vi "KPRO_2016_DPT.vi"() -> ()   [LabVIEW 2016]
uses:
  Kpro Globals.vi
  ad interface/Global_SIM_switch.vi
  <vilib>/Utility/file.llb/Write To Spreadsheet File (DBL).vi
panel:
  in  "Case Constant\n(See Context Help)":bool
  in  "Record DTW":bool
  out "Depth to Water":dbl=-30.877198474121087 format="%.2f"
  in  "In-Line Pressure Offset":dbl format="%.2f"
  in  "Zero In-Line Pressure\n(F = leave as is)":bool=TRUE
  in  "In-Line Pressure Slope":dbl=42.0 format="%.2f"
  out "In-Line Pressure":dbl=69.7228 format="%.2f"
  out "Drive Rate":dbl=16.666666666666664 format="%.2f"
  out "Real Time - Depth vs. Drive":cluster{dbl[], dbl[]}(graph)={[0.02036245163917736, 0.125, 0.16666666666666674, 0.16666666666666663, 0.16666666666666663, 0.16666666666666663], [-100.1, -100.2, -100.3, -100.4, -100.5, -100.6]}
  out "Current Depth (m)":sgl=-30.661383 format="%.2f"
  out "Zeroed \nPressure (m)":dbl=22.78027421497274 format="%.2f"
  out "Ik":dbl=0.003788962123473114 format="%.2f"
  in  "KPRO_test_report_header":string="Time(msecs)\tUncorrected_Depth\tCorrected_Depth\tDrive_Rate\tFlow\tFeet_of_Stainless\tPressure\tIK\tCorrected_Pressure\tAtm_Pressure\tDepth_to_water\tHeight_of_box\tRes_Pressure\tSecs_since_1_JAN_1904\tDepth_jumps_more_than_1_foot\r\n"
  in  "SLUG_test_report_header":string="Time(msecs)\tPressure\tFlow\n"
  in  "YSI_test_report_header":string="Depth\tPressure\tTemperature\tSpecific Conductivity\tDissolved O2\tPH\tOrp\tION\n"
  out "IK_for_GMS_report_header":string="Name\tHOLE_001\rXYZ\t20\t10\t30\rNumcols\t2\rNumrows\t1\rDepth\tIk\r"
  in  "Numrowswrite":string="1"
  in  "E":string="30"
  in  "Northing":string="10"
  in  "Easting":string="20"
  in  "Hole Id":string="HOLE_001"
  in  "Hole_name_file":path=path "C:/e"
  in  "Output File KPRO Test":path=path "C:/e_KPRO.txt"
  in  "Output File Slug Test":path=path "C:/e_SLUG.txt"
  in  "Output File YSI Test":path=path "C:/e_YSI.txt"
  in  "Output File IK for GMS":path=path "C:/e_IKMGS.txt"
  in  "enable_IKMGS_file":bool
  in  "enable_slug_file":bool
  in  "enable_kpro_file":bool=TRUE
  in  "enable_YSI_file":bool
  out "Ik":dbl=0.003788962123473114 format="%.2f"
  out "Zeroed Pressure":dbl=74.74207969932556 format="%.2f"
  out "Current Depth":sgl=-100.6 format="%.2f"
  out "Flow":dbl=0.21081600494384767 format="%.2f"
  out "Real Time - Depth vs. lk":cluster{dbl[], dbl[]}(graph)={[0.003788962123473114, 0.0037174584307500765, 0.0037174584307500765, 0.0037174584307500765, 0.0037174584307500765, 0.003788962123473114], [-100.1, -100.2, -100.3, -100.4, -100.5, -100.6]}
  out "Profile ID":string="WP-01"
  out "KPRO Box Number":dbl=800.0
  out "Last_String_Pot_Slope":dbl=1.6619999408721924 format="%.2f"
  out "Last_Flow_Slope":dbl=39.040000915527344 format="%.2f"
  out "Last_Pressure_Slope":dbl=48.27000045776367 format="%.2f"
  out "Height of Sample Box":dbl format="%.2f"
  out "Hole_Name_Path":path=path "C:/e"
  out "Cumulative_data_from_file":sgl[][](array[numeric]) format="%.2f"
  in  "data_directory":string="C:\\KPRO_DATA\\SITE_NAME\\"
  out "Cumulative_data_ready":bool
  out "Real Time - Depth vs. lk":cluster{dbl[], dbl[]}(graph)={[0.003788962123473114, 0.0037174584307500765, 0.0037174584307500765, 0.0037174584307500765, 0.0037174584307500765, 0.003788962123473114], [-100.1, -100.2, -100.3, -100.4, -100.5, -100.6]}
  in  "Reservoir Pressure":dbl=-0.004827000045779073 format="%.2f"
  in  "Simulate AD6B":bool
  in  "Atmospheric Pressure":dbl=32.22022530555725 format="%.2f"
  out "Depth to Water Table":dbl=-0.0 format="%.2f"
  in  "Ion Offset":dbl format="%.2f"
  in  "Ion Slope":dbl=44.04 format="%.2f"
  out "Pressure Slope":dbl=48.27000045776367 format="%.2f"
  out "Flow Slope":dbl=39.040000915527344 format="%.2f"
  out "String Pot Slope":dbl=1.6619999408721924 format="%.2f"
  in  "KPRO Com Port":i32=6
  in  "YSI Time Out (secs)":i32=5000
  in  "YSI Com Port":i32=7
  out "numrows":dbl format="%.2f"
  out "Slug Test\nIndicator copy":bool
  in  "ISE":bool=TRUE
  in  "Start\nYSI Capture":bool
  in  "Capture Head \nPressure":bool
  in  "Depth mode":bool caption="Use \nIncrement"
  out "Real Time - Depth vs. Drive":cluster{dbl[], dbl[]}(graph)={[0.02036245163917736, 0.125, 0.16666666666666674, 0.16666666666666663, 0.16666666666666663, 0.16666666666666663], [-100.1, -100.2, -100.3, -100.4, -100.5, -100.6]}
  out "Cumulative - Depth vs. Drive":cluster{dbl[], dbl[]}(graph)
  in  "Feet of Stainless":i32=40
  out "Zero Pressure\nIndicator":bool
  out "Slug Test\nIndicator":bool
  out "KPRO Test\nIndicator":bool
  in  "Increment\nButton":bool
  in  "Start\nST":bool
  in  "Zero\nPressure":bool
  out "Zeroed \nPressure":dbl=74.74207969932556 format="%.2f"
  in  "Finish Tests":bool
  out "Current Depth":sgl=-100.6 format="%.2f"
  in  "Start\nKPRO":bool
  out "Total Volume":dbl format="%.2f"
  in  "Clear \nTotal\nVolume":bool
  in  "Start Depth":sgl format="%.2f"
  in  "Client ID - Not Used":string
  out "Flow":dbl=0.21081600494384767 format="%.2f"
  out "Cumulative - Depth vs. Ik":cluster{dbl[], dbl[]}(graph)
  # "Use new slope/offset"
  # "KPRO  DATALOGGER"
  # "STONE  ENVIRONMENTAL  2010"
  # "ON"
  # "OFF"
  # "String Pot"
  # "Revision History\n\nAdded metric depth and pressure - VLD - 12-20-07\nAdded Static Ik button and drive rate- VLD 1-28-10"
  # "Use Incr"
  # "ON"
  # "OFF"
  # "ON"
  # "OFF"
  # "ON"
  # "OFF"
  # "ON"
  # "OFF"
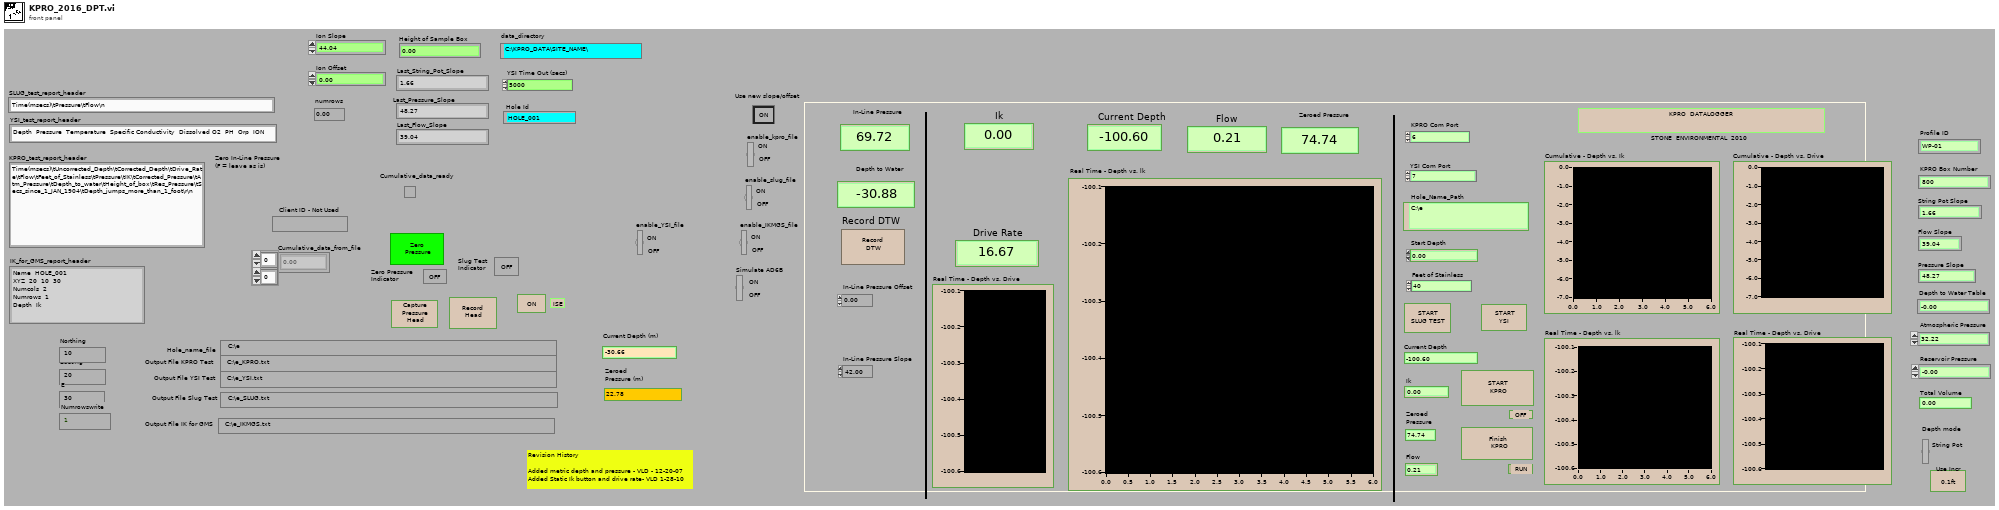
[diagram p1: front panel]
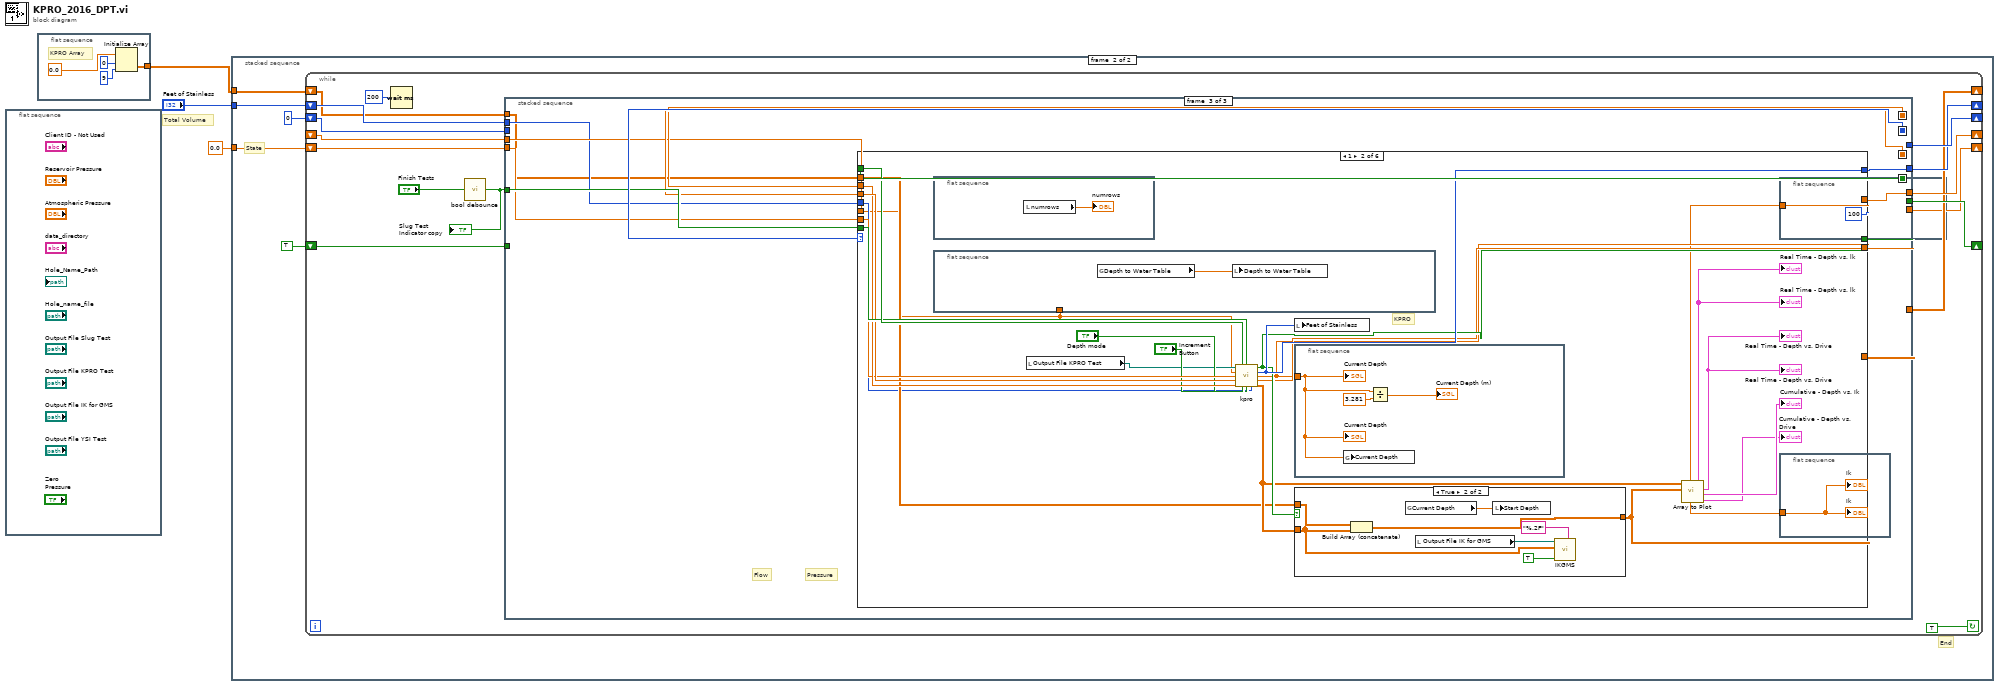
[diagram p0: block diagram]
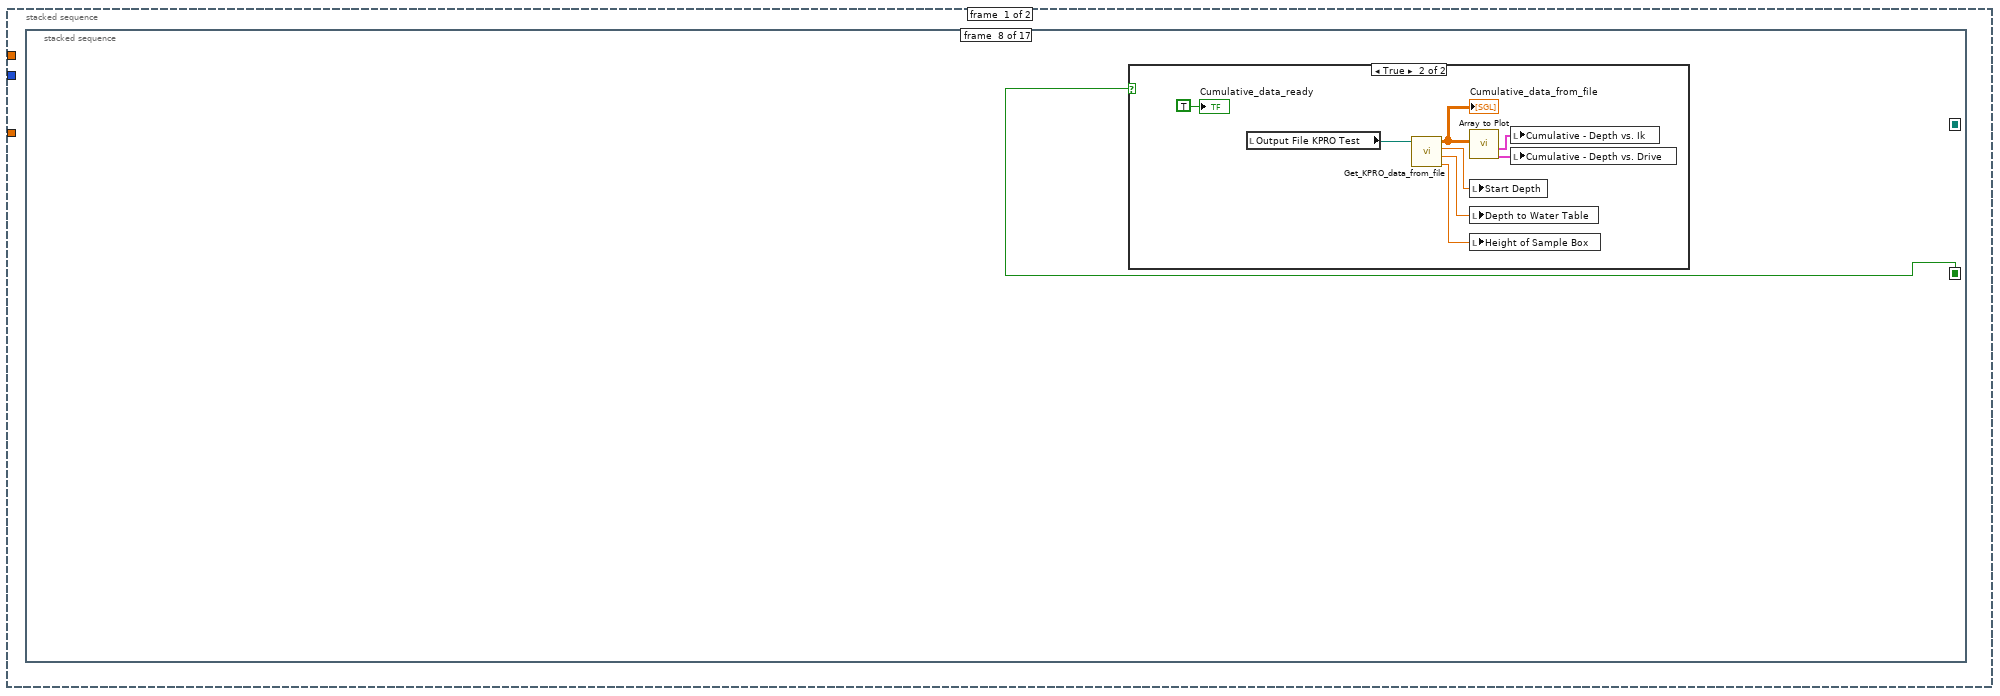
[diagram p2: hidden frame]
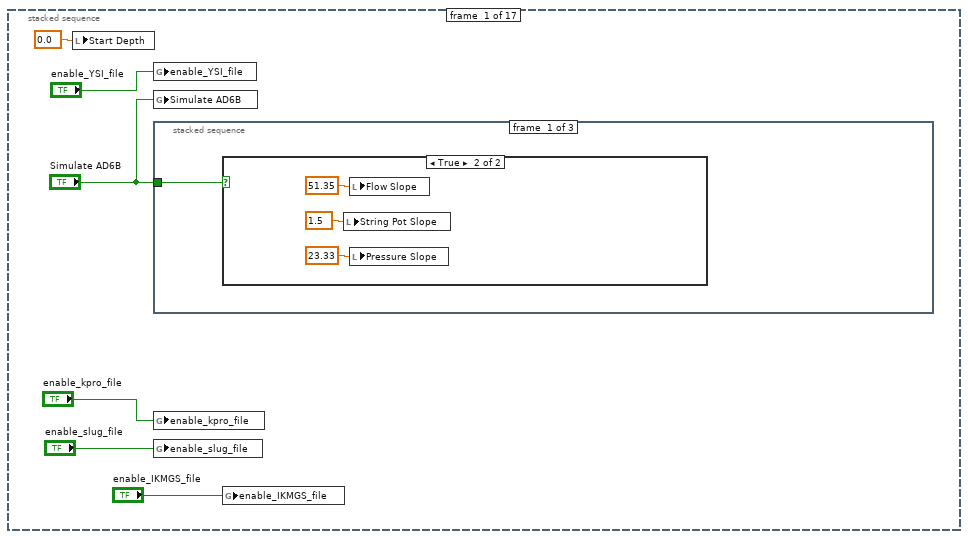
[diagram p3: hidden frame]
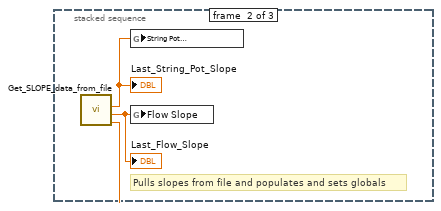
[diagram p5: hidden frame]
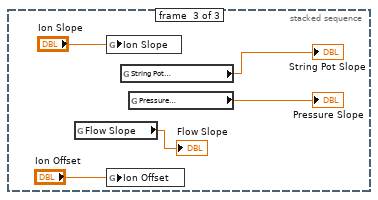
[diagram p6: hidden frame]
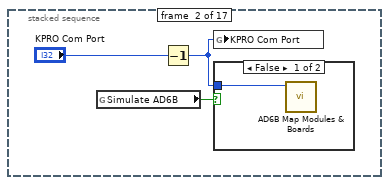
[diagram p7: hidden frame]
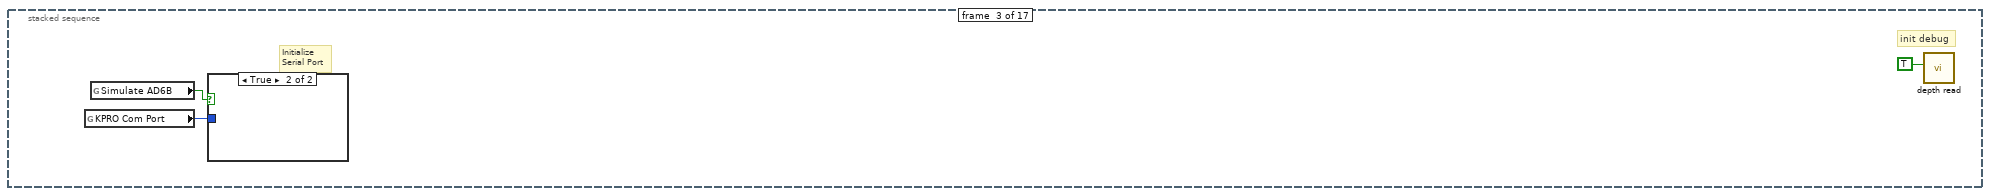
[diagram p9: hidden frame]
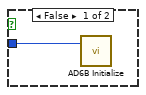
[diagram p10: hidden frame]
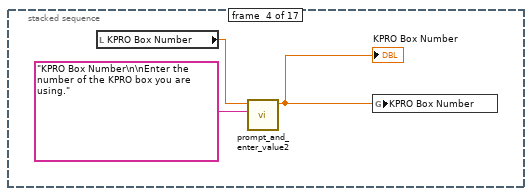
[diagram p11: hidden frame]
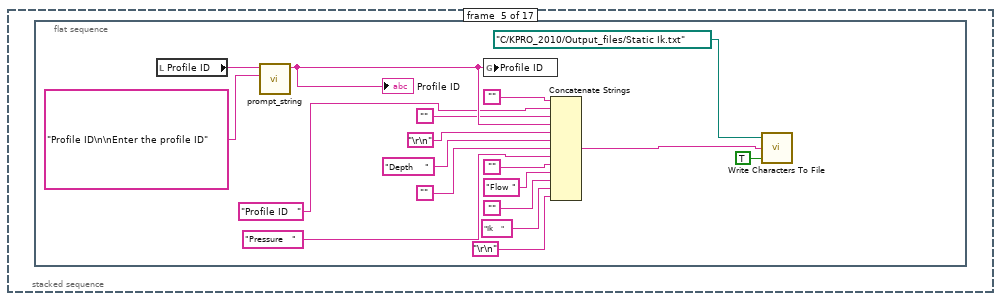
[diagram p12: hidden frame]
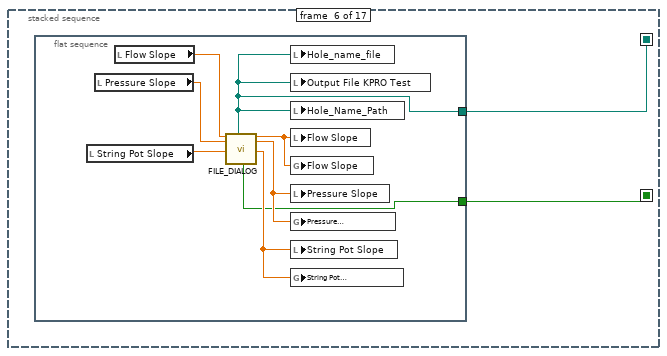
[diagram p13: hidden frame]
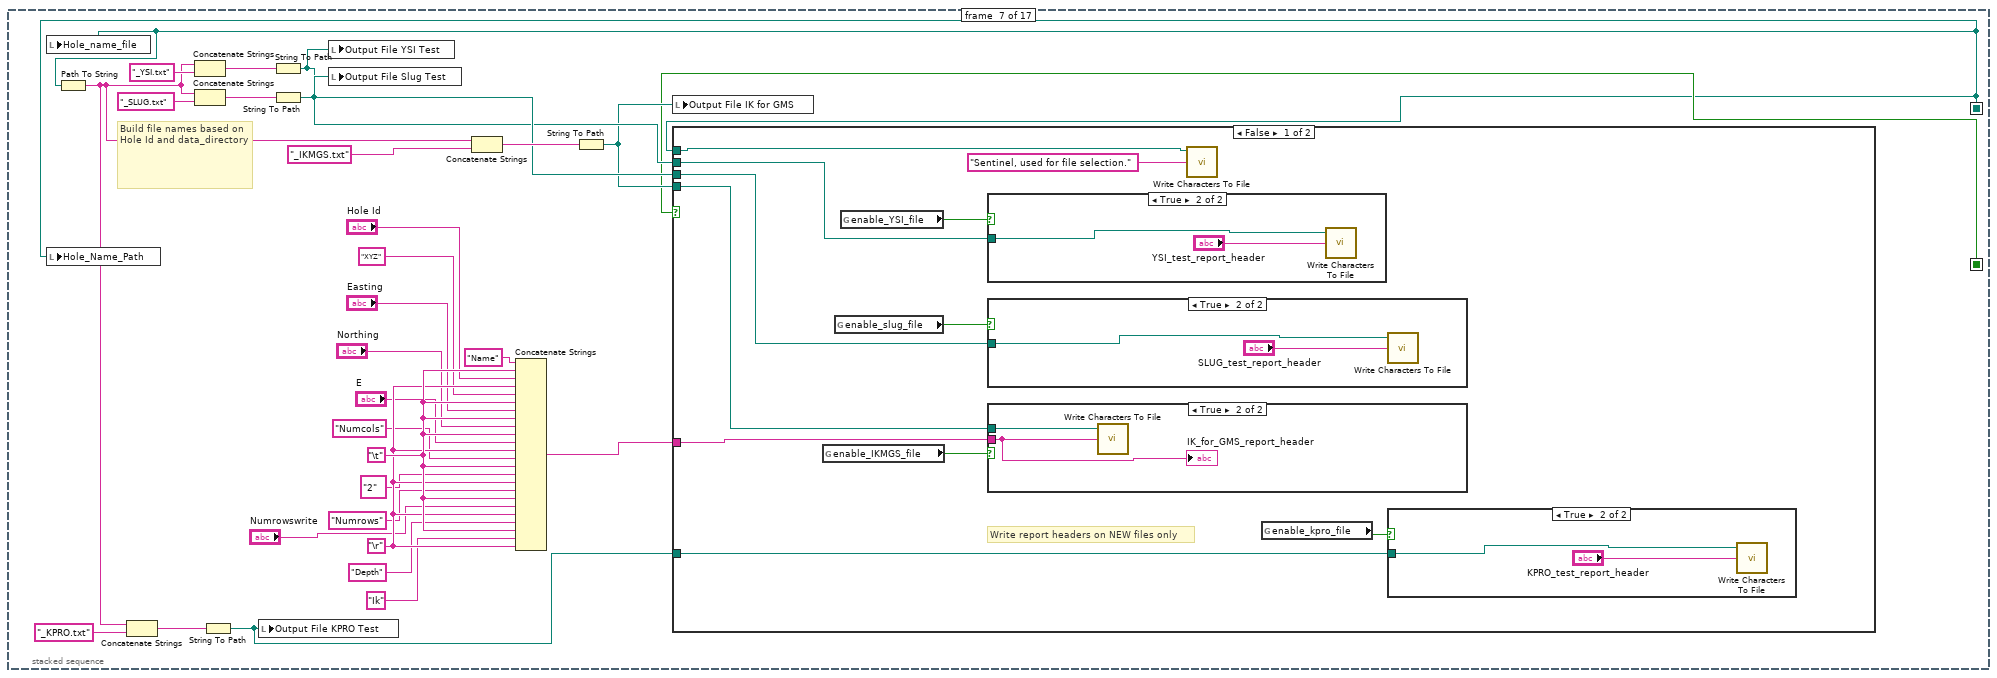
[diagram p14: hidden frame]
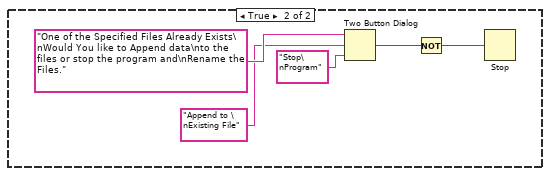
[diagram p19: hidden frame]
diagram:
  # "Total Volume"
  n1 = flat-sequence {
    frame #0 {
    }
  }
  n2 = flat-sequence {
    tunnel: [w4] -> w1
    frame #0 {
      # "KPRO Array"
      n3 = Initialize Array(0.0, 0, 9) -> (w4:dbl[][])
    }
  }
  n4 = stacked-sequence {
    tunnel: "Feet of Stainless" -> [_ w197]
    tunnel: 0.0 -> [_ w196]
    tunnel: w1 -> [_ w195]
    frame #0 {
      n5 = stacked-sequence {
        seq-local: [_ _ _ _ _ w55 _ _ _ _ _ _ _ _ _ _ _] -> [_ _ _ _ _ _ w66 w119 _ _ _ _ _ _ _ _ _]
        seq-local: [_ _ _ _ _ w56 _ _ _ _ _ _ _ _ _ _ _] -> [_ _ _ _ _ _ w65 _ _ _ _ _ _ _ _ _ _]
        frame #0 {
          n6 = local write "Start Depth"(sgl 0.0 ("Start Depth")) -> ()
          n7 = global write "Global_SIM_switch.vi" "enable_YSI_file"("enable_YSI_file") -> ()
          n8 = global write "Global_SIM_switch.vi" "Simulate AD6B"("Simulate AD6B") -> ()
          n9 = stacked-sequence {
            tunnel: "Simulate AD6B" -> [w14 _ _]
            frame #0 {
              n10 = case shown="True" w14 {
                frame False {
                }
                frame True {
                  n11 = local write "String Pot Slope"(1.5 ("String Pot Slope")) -> ()
                  n12 = local write "Flow Slope"(51.35 ("Flow Slope")) -> ()
                  n13 = local write "Pressure Slope"(23.33 ("Pressure Slope")) -> ()
                }
              }
            }
            frame #1 {
              # "Pulls slopes from file and populates and sets globals"
              n14 = call "Get_SLOPE_data_from_file.vi"() -> ("Last_Pressure_Slope"=w20:dbl, "Last_Flow_Slope"=w19:dbl, "Last_String_Pot_Slope"=w18:dbl)  [unwired: 8 in, 1 out]
              "Last_Pressure_Slope" <- w20
              "Last_Flow_Slope" <- w19
              "Last_String_Pot_Slope" <- w18
              n15 = global write "Kpro Globals.vi" "String Pot \nSlope"(w18) -> ()
              n16 = global write "Kpro Globals.vi" "Flow Slope"(w19) -> ()
              n17 = global write "Kpro Globals.vi" "Pressure \nSlope"(w20) -> ()
            }
            frame #2 {
              n18 = global read "Kpro Globals.vi" "Flow Slope"() -> (→"Flow Slope":dbl)
              n19 = global write "Kpro Globals.vi" "Ion Slope"("Ion Slope") -> ()
              n20 = global write "Kpro Globals.vi" "Ion Offset"("Ion Offset") -> ()
              n21 = global read "Kpro Globals.vi" "String Pot \nSlope"() -> (→"String Pot Slope":dbl)
              n22 = global read "Kpro Globals.vi" "Pressure \nSlope"() -> (→"Pressure Slope":dbl)
            }
          }
          n23 = global write "Global_SIM_switch.vi" "enable_kpro_file"("enable_kpro_file") -> ()
          n24 = global write "Global_SIM_switch.vi" "enable_slug_file"("enable_slug_file") -> ()
          n25 = global write "Global_SIM_switch.vi" "enable_IKMGS_file"("enable_IKMGS_file") -> ()
        }
        frame #1 {
          n26 = global read "Global_SIM_switch.vi" "Simulate AD6B"() -> (w26:bool)
          n27 = Decrement(x="KPRO Com Port") -> (x-1=w27:i32)
          n28 = global write "Kpro Globals.vi" "KPRO Com Port"(w27) -> ()
          n29 = case shown="False" w26 {
            tunnel: w27 -> [w29 _]
            frame False {
              n30 = call "AD6B Map Modules & Boards.VI"("port number (1:com2)"=w29) -> ()  [unwired: 3 in, 3 out]
            }
            frame True {
            }
          }
        }
        frame #2 {
          # "init debug"
          # "Initialize\nSerial Port"
          n31 = global read "Kpro Globals.vi" "KPRO Com Port"() -> (w30:i32)
          n32 = global read "Global_SIM_switch.vi" "Simulate AD6B"() -> (w31:bool)
          n33 = case shown="True" w31 {
            tunnel: w30 -> [w33 _]
            frame False {
              n34 = call "AD6B Initialize.VI"("port number (1:com2)"=w33) -> ()  [unwired: 2 in, 1 out]
            }
            frame True {
            }
          }
          n35 = call "depth read.vi"("Initialize Debug"=TRUE) -> ()  [unwired: 3 in, 1 out]
        }
        frame #3 {
          n36 = local read "KPRO Box Number"() -> (w34:dbl)
          n37 = call "prompt_and_enter_value2.vi"("prompt_IN"="KPRO Box Number\n\nEnter the number of the KPRO box you are using." ("prompt"), "Enter value"=w34) -> ("Numeric"=w35:dbl)  [unwired: 9 in]
          "KPRO Box Number" <- w35
          n38 = global write "Kpro Globals.vi" "KPRO Box Number"(w35) -> ()
        }
        frame #4 {
          n39 = flat-sequence {
            frame #0 {
              n40 = local read "Profile ID"() -> (w54:string)
              n41 = call "prompt_string.vi"("prompt_IN"="Profile ID\n\nEnter the profile ID" ("prompt"), "Enter value"=w54) -> ("String"=w50:string)  [unwired: 9 in]
              "Profile ID" <- w50
              n42 = global write "Kpro Globals.vi" "Profile ID"(w50) -> ()
              n43 = Concatenate Strings("" ("string"), "Profile ID   " ("string"), "" ("string"), w50, "\r\n", "Depth    " ("string"), "" ("string"), "Pressure   " ("string"), "" ("string"), "Flow " ("string"), "" ("string"), "Ik    " ("string"), "\r\n") -> (w49:string)
              n44 = call <vilib>:"Write Characters To File.vi"("append to file? (new file:F)"=TRUE, "character string"=w49, "file path (dialog if empty)"=path "C:/KPRO_2010/Output_files/Static Ik.txt") -> ()  [unwired: 2 in, 1 out]
            }
          }
        }
        frame #5 {
          n45 = flat-sequence {
            tunnel: [w58] -> w56
            tunnel: [w57] -> w55
            frame #0 {
              n46 = local read "String Pot Slope"() -> (w62:dbl)
              n47 = local read "Pressure Slope"() -> (w63:dbl)
              n48 = local read "Flow Slope"() -> (w64:dbl)
              n49 = call "FILE_DIALOG.vi"("flow_slope_IN"=w64, "pressure_slope_IN"=w63, "string_pot_slope_IN"=w62) -> ("path"=w58:path, "exists"=w57:bool, "flow_slope_OUT"=w61:dbl, "pressure_slope_OUT"=w60:dbl, "string_pot_slope_OUT"=w59:dbl)  [unwired: 9 in, 3 out]
              n50 = local write "Hole_name_file"(w58) -> ()
              n51 = local write "Output File KPRO Test"(w58) -> ()
              n52 = local write "Hole_Name_Path"(w58) -> ()
              n53 = local write "Flow Slope"(w61) -> ()
              n54 = global write "Kpro Globals.vi" "Flow Slope"(w61) -> ()
              n55 = local write "Pressure Slope"(w60) -> ()
              n56 = global write "Kpro Globals.vi" "Pressure \nSlope"(w60) -> ()
              n57 = local write "String Pot Slope"(w59) -> ()
              n58 = global write "Kpro Globals.vi" "String Pot \nSlope"(w59) -> ()
            }
          }
        }
        frame #6 {
          w94 = "\t"
          w93 = "\r" ("Carriage Return")
          # "Build file names based on Hole Id and data_directory"
          n59 = local write "Hole_name_file"(w65) -> ()
          n60 = local write "Hole_Name_Path"(w65) -> ()
          n61 = Path To String(path=w65) -> (string=w76:string)
          n62 = Concatenate Strings(w76, "_KPRO.txt") -> (w82:string)
          n63 = Concatenate Strings(w76, "_YSI.txt") -> (w80:string)
          n64 = Concatenate Strings(w76, "_SLUG.txt") -> (w81:string)
          n65 = String To Path(string=w82) -> (path=w75:path)
          n66 = local write "Output File KPRO Test"(w75) -> ()
          n67 = String To Path(string=w80) -> (path=w73:path)
          n68 = String To Path(string=w81) -> (path=w74:path)
          n69 = local write "Output File YSI Test"(w73) -> ()
          n70 = local write "Output File Slug Test"(w74) -> ()
          n71 = Concatenate Strings(w76, "_IKMGS.txt") -> (w79:string)
          n72 = Concatenate Strings("Name" ("Name"), w94, "Hole Id", w93, "XYZ" ("date string"), w94, "Easting", w94, "Northing", w94, "E", w93, "Numcols", w94, "2", w93, "Numrows", w94, "Numrowswrite", w93, "Depth", w94, "Ik", w93) -> (w85:string)
          n73 = String To Path(string=w79) -> (path=w72:path)
          n74 = local write "Output File IK for GMS"(w72) -> ()
          n75 = case shown="False" w66 {
            tunnel: w85 -> [w99 _]
            tunnel: w65 -> [w104 _]
            tunnel: w75 -> [w103 _]
            tunnel: w74 -> [w102 _]
            tunnel: w73 -> [w101 _]
            tunnel: w72 -> [w100 _]
            frame False {
              # "Write report headers on NEW files only"
              n76 = global read "Global_SIM_switch.vi" "enable_IKMGS_file"() -> (w95:bool)
              n77 = global read "Global_SIM_switch.vi" "enable_slug_file"() -> (w97:bool)
              n78 = global read "Global_SIM_switch.vi" "enable_YSI_file"() -> (w96:bool)
              n79 = case shown="True" w96 {
                tunnel: w101 -> [_ w109]
                frame False {
                }
                frame True {
                  n80 = call <vilib>:"Write Characters To File.vi"("character string"="YSI_test_report_header", "file path (dialog if empty)"=w109) -> ()  [unwired: 3 in, 1 out]
                }
              }
              n81 = case shown="True" w97 {
                tunnel: w102 -> [_ w111]
                frame False {
                }
                frame True {
                  n82 = call <vilib>:"Write Characters To File.vi"("character string"="SLUG_test_report_header", "file path (dialog if empty)"=w111) -> ()  [unwired: 3 in, 1 out]
                }
              }
              n83 = case shown="True" w95 {
                tunnel: w100 -> [_ w107]
                tunnel: w99 -> [_ w106]
                frame False {
                }
                frame True {
                  n84 = call <vilib>:"Write Characters To File.vi"("character string"=w106, "file path (dialog if empty)"=w107) -> ()  [unwired: 3 in, 1 out]
                  "IK_for_GMS_report_header" <- w106
                }
              }
              n85 = call <vilib>:"Write Characters To File.vi"("character string"="Sentinel, used for file selection.", "file path (dialog if empty)"=w104) -> ()  [unwired: 3 in, 1 out]
              n86 = global read "Global_SIM_switch.vi" "enable_kpro_file"() -> (w98:bool)
              n87 = case shown="True" w98 {
                tunnel: w103 -> [_ w113]
                frame False {
                }
                frame True {
                  n88 = call <vilib>:"Write Characters To File.vi"("character string"="KPRO_test_report_header", "file path (dialog if empty)"=w113) -> ()  [unwired: 3 in, 1 out]
                }
              }
            }
            frame True {
              n89 = Two Button Dialog(message="One of the Specified Files Already Exists\nWould You like to Append data\nto the files or stop the program and\nRename the Files.", 1:"Stop\nProgram", 2:"Append to \nExisting File") -> (T button?=w114:bool)
              n90 = Not(x=w114) -> (.not. x?=w115:bool)
              n91 = Stop(stop? (T)=w115) -> ()
            }
          }
        }
        frame #7 {
          n92 = case shown="True" w119 {
            frame False {
            }
            frame True {
              n93 = local read "Output File KPRO Test"() -> (w123:path)
              n94 = call "Get_KPRO_data_from_file.vi"("Output File KPRO Test"=w123) -> ("Last_height_of_box"=w120:dbl, "Last_depth_to_water"=w121:dbl, "Last_depth"=w127:dbl, "Output_array"=w124:sgl[][])  [unwired: 7 in]
              "Cumulative_data_from_file" <- w124
              n95 = call "Array to Plot.vi"("Input Cumulative Array"=w124) -> ("Cumulative - Depth vs.Drive Rate"=w125:cluster{dbl[], dbl[]}, "Cumulative - Depth vs. Ik"=w126:cluster{dbl[], dbl[]})  [unwired: 3 in, 4 out]
              n96 = local write "Start Depth"(w127) -> ()
              n97 = local write "Depth to Water Table"(w121) -> ()
              n98 = local write "Height of Sample Box"(w120) -> ()
              n99 = local write "Cumulative - Depth vs. Ik"(w126) -> ()
              n100 = local write "Cumulative - Depth vs. Drive"(w125) -> ()
              "Cumulative_data_ready" <- TRUE ("Cumulative_data_ready")
            }
          }
        }
        frame #8 {
          # "Start with Zero Offset for measurement of absolute pressure."
          n101 = global read "Global_SIM_switch.vi" "Simulate AD6B"() -> (w128:bool)
          n102 = case shown="False" w128 {
            tunnel: TRUE -> [w131 w133]
            tunnel: 0.0 -> [w132 w134]
            frame False {
              n103 = call "Pressure.vi"("Zero Pressure\n(F = leave as is)"=w131, "Pressure Offset"=w132) -> ()  [unwired: 1 in, 1 out]
            }
            frame True {
              n104 = call "SIM_Pressure.vi"("Zero Pressure\n(F = leave as is)"=w133, "Pressure Offset"=w134) -> ()  [unwired: 9 in, 1 out]
            }
          }
        }
        frame #9 {
          # "Take offset and put\n into Pressure VI."
          n105 = call "PRESSURE_CAL.vi"("sim_low"=29.9 ("sim_high"), "sim_high"=29.96, "Prompt_IN"="ATMOSPHERIC PRESSURE READING\n\nHold Kpro effluent facing up and level with the pressure transducer.\nTurn on Kpro water, turn off when water flows with no air bubbles.\n\nPress OK when the reading equilibrates." ("message")) -> ("PRESSURE\nFt of water"=w135:dbl)  [unwired: 8 in]
          n106 = global read "Global_SIM_switch.vi" "Simulate AD6B"() -> (w136:bool)
          n107 = global write "Kpro Globals.vi" "Atmospheric Pressure"(w135) -> ()
          n108 = local write "Atmospheric Pressure"(w135) -> ()
          n109 = case shown="False" w136 {
            tunnel: w135 -> [w142 w144]
            tunnel: TRUE -> [w141 w143]
            frame False {
              n110 = call "Pressure.vi"("Zero Pressure\n(F = leave as is)"=w141, "Pressure Offset"=w142) -> ()  [unwired: 1 in, 1 out]
            }
            frame True {
              n111 = call "SIM_Pressure.vi"("Zero Pressure\n(F = leave as is)"=w143, "Pressure Offset"=w144) -> ()  [unwired: 9 in, 1 out]
            }
          }
        }
        frame #10 {
          n112 = case shown="True" "Case Constant\n(See Context Help)" {
            frame False {
            }
            frame True {
              # "Take offset and put\n into Pressure VI."
              n113 = call "PRESSURE_CAL.vi"("sim_low"=30.9 ("sim_high"), "sim_high"=30.96, "Prompt_IN"="ZERO PRESSURE TRANSDUCER\n\nHold Kpro effluent in a grad cylinder with 800mL (1 ft) of water.\nHold grad cylinder with its bottom level with the pressure transducer.\n\nPress OK when the reading equilibrates. " ("message")) -> ("PRESSURE\nFt of water"=w146:dbl)  [unwired: 8 in]
              n114 = global read "Global_SIM_switch.vi" "Simulate AD6B"() -> (w148:bool)
              n115 = Subtract(x=w146, y=1.0) -> (x-y=w150:dbl)
              n116 = case shown="False" w148 {
                tunnel: [w155 w156] -> w149
                frame False {
                  n117 = call "Flow.vi"() -> ("Flow (ml/min)"=w155:dbl)  [unwired: 3 in]
                }
                frame True {
                  n118 = call "SIM_Flow.vi"() -> ("Flow (ml/min)"=w156:dbl)  [unwired: 3 in]
                }
              }
              n119 = case shown="False" w148 {
                tunnel: w150 -> [w158 w160]
                tunnel: TRUE -> [w157 w159]
                frame False {
                  n120 = call "Pressure.vi"("Zero Pressure\n(F = leave as is)"=w157, "Pressure Offset"=w158) -> ()  [unwired: 1 in, 1 out]
                }
                frame True {
                  n121 = call "SIM_Pressure.vi"("Zero Pressure\n(F = leave as is)"=w159, "Pressure Offset"=w160) -> ()  [unwired: 9 in, 1 out]
                }
              }
              n122 = local write "Flow"(w149) -> ()
            }
          }
        }
        frame #11 {
          n123 = call "PRESSURE_CAL.vi"("sim_low"=99.5 ("sim_high"), "sim_high"=100.5, "Prompt_IN"="CHECK RESERVOIR PRESSURE\n\nTurn on Kpro. Unplug Kpro Out quick connect from sample box.\nReservoir pressure should be 69.2 +/- 5%(65.7 - 72.7).\n\nPress OK when the reading equilibrates within range." ("message")) -> ("PRESSURE\nFt of water"=w163:dbl)  [unwired: 8 in]
          n124 = local write "Reservoir Pressure"(w163) -> ()
          n125 = global write "Kpro Globals.vi" "Reservoir Pressure"(w163) -> ()
        }
        frame #12 {
          n126 = local read "Start Depth"() -> (w169:sgl)
          n127 = call "prompt_and_enter_value 2016.vi"("prompt_IN"="ENTER START DEPTH", "Enter value"=w169) -> ("Numeric"=w167:dbl)  [unwired: 9 in]
          n128 = Absolute Value(x=w167) -> (abs(x)=w166:dbl)
          n129 = Negate(x=w166) -> (-x=w165:dbl)
          n130 = local write "Start Depth"(w165) -> ()
        }
        frame #13 {
          n131 = local read "Height of Sample Box"() -> (w171:dbl)
          n132 = call "prompt_and_enter_value 2016.vi"("prompt_IN"="HEIGHT FROM GROUND SURFACE TO SAMPLE BOX\n\nMeasure the vertical distance between the ground surface and the pressure transducer." ("prompt"), "Enter value"=w171) -> ("Numeric"=w170:dbl)  [unwired: 9 in]
          "Height of Sample Box" <- w170
          n133 = global write "Kpro Globals.vi" "height_of_box"(w170) -> ()
        }
        frame #14 {
          n134 = flat-sequence {
            frame #0 {
              n135 = local read "Depth to Water Table"() -> (w176:dbl)
              n136 = call "prompt_and_enter_value 2016.vi"("prompt_IN"="DEPTH TO WATER TABLE\n\nEnter the depth to the water table." ("prompt"), "Enter value"=w176) -> ("Numeric"=w175:dbl)  [unwired: 9 in]
              n137 = Absolute Value(x=w175) -> (abs(x)=w174:dbl)
              n138 = Negate(x=w174) -> (-x=w173:dbl)
              "Depth to Water Table" <- w173
              n139 = global write "Kpro Globals.vi" "Depth to Water Table"(w173) -> ()
            }
          }
        }
        frame #15 {
          n140 = stacked-sequence {
            frame #0 {
              # "Set to raw pressure mode"
              n141 = global read "Global_SIM_switch.vi" "Simulate AD6B"() -> (w179:bool)
              n142 = case shown="False" w179 {
                tunnel: TRUE -> [w180 w182]
                frame False {
                  n143 = call "Pressure.vi"("Zero Pressure\n(F = leave as is)"=w180, "Pressure Offset"=0.0) -> ()  [unwired: 1 in, 1 out]
                }
                frame True {
                  n144 = call "SIM_Pressure.vi"("Zero Pressure\n(F = leave as is)"=w182) -> ()  [unwired: 10 in, 1 out]
                }
              }
            }
            frame #1 {
              # "adjust for 1 foot head"
              # "Take offset and put\n into Pressure VI."
              n145 = global read "Global_SIM_switch.vi" "Simulate AD6B"() -> (w186:bool)
              n146 = call "PRESSURE_CAL.vi"("sim_low"=29.9 ("sim_high"), "sim_high"=29.96, "Prompt_IN"="ZERO TO GROUND SURFACE\n\nFill a grad cylinder to 750mL.\nPlace it on the ground at the profile location.\nImmerse the Kpro effluent and turn on Kpro flow.\nTurn off after water is flowing with no bubbles\nand the water has reached 800mL (1 foot).\n\nPress OK when the reading equilibrates." ("message")) -> ("PRESSURE\nFt of water"=w183:dbl)  [unwired: 8 in]
              n147 = Decrement(x=w183) -> (x-1=w184:dbl)
              n148 = case shown="False" w186 {
                tunnel: w184 -> [w191 w193]
                tunnel: TRUE -> [w190 w192]
                frame False {
                  n149 = call "Pressure.vi"("Zero Pressure\n(F = leave as is)"=w190, "Pressure Offset"=w191) -> ()  [unwired: 1 in, 1 out]
                }
                frame True {
                  n150 = call "SIM_Pressure.vi"("Zero Pressure\n(F = leave as is)"=w192, "Pressure Offset"=w193) -> ()  [unwired: 9 in, 1 out]
                }
              }
            }
          }
        }
        frame #16 {
          n151 = flat-sequence {
            frame #0 {
              w194 = FALSE
              n152 = local write "Slug Test\nIndicator"(w194) -> ()
              n153 = local write "KPRO Test\nIndicator"(w194) -> ()
              "Zero Pressure\nIndicator" <- w194
            }
          }
        }
      }
    }
    frame #1 {
      # "End"
      # "State"
      n154 = while {
        shift-left: w195 -> [w206]
        shift-right: [w205] -> _
        shift-left: w197 -> [w208]
        shift-right: [w207] -> _
        shift-left: _ -> [w211]
        shift-right: [w210] -> _
        shift-left: w196 -> [w209]
        shift-right: [w204] -> _
        shift-left: TRUE -> [w214]
        shift-right: [w213] -> _
        shift-left: 0 -> [w215]
        shift-right: [w212] -> _
        stop <- TRUE continue-if-true
        n155 = Wait (ms)(milliseconds to wait=u32 200) -> ()  [unwired: 1 out]
        n156 = call "bool debounce.vi"("Input Boolean"="Finish Tests") -> ("Output Boolean"=w202:bool)
        "Slug Test\nIndicator copy" <- w202
        n157 = stacked-sequence {
          seq-local: [_ w245 _] -> [_ _ w277]
          seq-local: [_ w256 _] -> [_ _ w276]
          seq-local: [w223 _ _] -> [_ _ w274]
          seq-local: [w224 _ _] -> [_ _ w273]
          tunnel: w215 -> [_ w258 _]
          tunnel: w214 -> [_ w257 _]
          tunnel: [_ _ w278] -> w213
          tunnel: [_ w245 _] -> w212
          tunnel: w202 -> [_ _ w275]
          tunnel: w211 -> [_ _ w272]
          tunnel: [_ _ w271] -> w210
          tunnel: w209 -> [_ _ w270]
          tunnel: [_ _ w269] -> w204
          tunnel: w208 -> [_ _ w268]
          tunnel: [_ _ w267] -> w207
          tunnel: w206 -> [_ _ w266]
          tunnel: [_ _ w265] -> w205
          frame #0 {
            n158 = global read "Kpro Globals.vi" "Current Depth"() -> (w219:sgl)
            n159 = call "In-Line-Pressure.vi"("Zero Pressure\n(F = leave as is)"="Zero In-Line Pressure\n(F = leave as is)", "In-Line Pressure Slope"="In-Line Pressure Slope", "In-Line Pressure Offset"="In-Line Pressure Offset") -> ("Pressure"=w220:dbl)  [unwired: 1 in]
            "In-Line Pressure" <- w220
            n160 = Add(x=w220, y=w219) -> (x+y=w216:dbl)
            "Depth to Water" <- w216
            n161 = case shown="True" "Record DTW" {
              selector: "Record DTW" -> [w230 _]
              tunnel: [w230 FALSE ("Boolean")] -> _
              tunnel: w216 -> [_ w234]
              tunnel: w219 -> [_ w235]
              tunnel: "In-Line Pressure Offset" -> [_ w232]
              tunnel: w220 -> [_ w233]
              tunnel: "In-Line Pressure Slope" -> [_ w231]
              frame False {
              }
              frame True {
                n162 = Build Array(w235, w234, w233, w232, w231) -> (w239:dbl[])
                n163 = call-poly <vilib>:"Write To Spreadsheet File.vi"("append to file? (new file:F)"=TRUE, "1D data"=w239, "file path (dialog if empty)"=path "C:/KPRO_2010/Output_files/DTW.txt") -> ()  [unwired: 5 in, 1 out]
              }
            }
            n164 = global read "Global_SIM_switch.vi" "Simulate AD6B"() -> (w225:bool)
            n165 = case shown="False" w225 {
              tunnel: [w242 w244] -> w224
              tunnel: [w241 w243] -> w223
              frame False {
                n166 = call "Flow.vi"() -> ("Flow (ml/min)"=w242:dbl)  [unwired: 3 in]
                n167 = call "Pressure.vi"("Zero Pressure\n(F = leave as is)"=FALSE ("Zero Pressure\n(F = leave as is)")) -> ("Pressure"=w241:dbl)  [unwired: 2 in]
              }
              frame True {
                n168 = call "SIM_Flow.vi"() -> ("Flow (ml/min)"=w244:dbl)  [unwired: 3 in]
                n169 = call "SIM_Pressure.vi"() -> ("Pressure"=w243:dbl)  [unwired: 11 in]
              }
            }
            n170 = flat-sequence {
              tunnel: w224 -> [w226]
              frame #0 {
                "Flow" <- w226
                "Flow" <- w226
              }
            }
            n171 = flat-sequence {
              tunnel: w223 -> [w229]
              frame #0 {
                n172 = Divide(x=w229, y=3.281) -> (x/y=→"Zeroed \nPressure (m)":dbl)
                "Zeroed \nPressure" <- w229
                "Zeroed Pressure" <- w229
              }
            }
          }
          frame #1 {
            n173 = call "State Controller.vi"("Start KPRO"="Start\nKPRO", "Start Slug Test"="Start\nST", "Start YSI Capture"="Start\nYSI Capture", "Clear Volume"="Clear \nTotal\nVolume", "Capture Head Pressure"="Capture Head \nPressure", "Done"=w257, "Previous \nState"=w258) -> ("Next State"=w245:i32, "State Changed"=w256:bool, "Start KPRO Enabler"=w250:u8, "Start Slug Test Enabler"=w249:u8, "Start YSI Capture Enabler"=w248:u8, "Clear Volume Enabler"=w247:u8, "Capture Head Pressure Enabler"=w246:u8)  [unwired: 4 in, 2 out]
            n174 = property on="Start\nKPRO" class="Bool"("Disabled"=w250) -> ()  [unwired: 2 in, 2 out]
            n175 = property on="Start\nST" class="Bool"("Disabled"=w249) -> ()  [unwired: 2 in, 2 out]
            n176 = property on="Clear \nTotal\nVolume" class="Bool"("Disabled"=w247) -> ()  [unwired: 2 in, 2 out]
            n177 = flat-sequence {
              tunnel: w245 -> [w259]
              frame #0 {
                n178 = Equal?(x=w259, y=2) -> (x = y?=→"Slug Test\nIndicator":bool)
              }
            }
            n179 = flat-sequence {
              tunnel: w245 -> [w262]
              frame #0 {
                n180 = Equal?(x=w262, y=1) -> (x = y?=→"KPRO Test\nIndicator":bool)
              }
            }
            n181 = property on="Start\nYSI Capture" class="Bool"("Disabled"=w248) -> ()  [unwired: 2 in, 2 out]
            n182 = property on="Capture Head \nPressure" class="Bool"("Disabled"=w246) -> ()  [unwired: 2 in, 2 out]
          }
          frame #2 {
            # "Flow"
            # "Pressure"
            n183 = case shown="1" w277 {
              tunnel: [FALSE w307 w333 w340 TRUE TRUE] -> w278
              tunnel: w276 -> [_ w315 w333 w342 _ _]
              tunnel: w275 -> [_ w314 _ w341 _ _]
              tunnel: w274 -> [_ w313 _ _ _ w361]
              tunnel: w273 -> [_ w312 _ _ _ _]
              tunnel: w272 -> [_ w293 w334 w343 w358 w360]
              tunnel: [w279 w297 w334 w343 w358 w360] -> w271
              tunnel: w270 -> [w284 w311 w337 w346 _ w365]
              tunnel: [w284 w302 w337 w346 0.0 w365] -> w269
              tunnel: w268 -> [w283 w294 w335 w345 w356 w364]
              tunnel: [w283 w308 w335 w345 w356 w364] -> w267
              tunnel: w266 -> [w282 w301 w336 w344 w355 w363]
              tunnel: [w281 w305 w336 w344 w355 w363] -> w265
              frame 0, Default {
                # "Idle State"
                n184 = local read "Cumulative_data_ready"() -> (w280:bool)
                n185 = case shown="True" w280 {
                  tunnel: w282 -> [w290 _]
                  tunnel: [w290 w291] -> w281
                  frame False {
                  }
                  frame True {
                    n186 = local read "Cumulative_data_from_file"() -> (w291:sgl[][])
                    n187 = local write "Cumulative_data_ready"(FALSE ("Get_KPRO_data")) -> ()
                  }
                }
                n188 = flat-sequence {
                  tunnel: [w286] -> w279
                  frame #0 {
                    n189 = Less Or Equal To 0?(x="Start Depth") -> (x <= 0?=w289:bool)
                    n190 = Negate(x="Start Depth") -> (-x=w287:sgl)
                    n191 = Select(t="Start Depth", s=w289, f=w287) -> (s? t:f=w286:sgl)
                  }
                }
              }
              frame 1 {
                # "KPRO"
                n192 = flat-sequence {
                  frame #0 {
                    n193 = local read "numrows"() -> (→"numrows":dbl)
                  }
                }
                n194 = flat-sequence {
                  tunnel: w293 -> [_]
                  frame #0 {
                    n195 = global read "Kpro Globals.vi" "Depth to Water Table"() -> (w317:dbl)
                    n196 = local write "Depth to Water Table"(w317) -> ()
                  }
                }
                n197 = local read "Output File KPRO Test"() -> (w300:path)
                n198 = call "kpro.vi"("Output KPRO"=w300, "Initialize"=w315, "Finished In"=w314, "Absolute Depth In"=w293, "Total Volume in"=w311, "Zeroed Pressure"=w313, "Flow"=w312, "Read String Pot"="Depth mode", "Increment"="Increment\nButton", "SS In"=w294) -> ("Finished Out"=w307:bool, "SS Out"=w308:i32, "Current Depth Out"=w297:sgl, "Total Volume Out"=w302:dbl, "Output Array"=w306:dbl[][])  [unwired: 1 in]
                n199 = local write "Feet of Stainless"(w308) -> ()
                n200 = flat-sequence {
                  tunnel: w297 -> [w320]
                  frame #0 {
                    n201 = global write "Kpro Globals.vi" "Current Depth"(w320) -> ()
                    n202 = Divide(x=w320, y=3.281) -> (x/y=→"Current Depth (m)":dbl)
                    "Current Depth" <- w320
                    "Current Depth" <- w320
                  }
                }
                n203 = case shown="True" w307 {
                  tunnel: [w325 w332] -> w305
                  tunnel: w306 -> [_ w331]
                  tunnel: w301 -> [w325 w327]
                  frame False {
                  }
                  frame True {
                    n204 = Build Array (concatenate)(w327, w331) -> (w332:dbl[][])
                    n205 = global read "Kpro Globals.vi" "Current Depth"() -> (w326:sgl)
                    n206 = local read "Output File IK for GMS"() -> (w329:path)
                    n207 = local write "Start Depth"(w326) -> ()
                    n208 = call "IKGMS.vi"("format (%.3f)"="%.2F", "append to file? (new file:F)"=TRUE, "2D data"=w331, "file path (dialog if empty)"=w329) -> ()  [unwired: 4 in, 1 out]
                  }
                }
                n209 = call "Array to Plot.vi"("Input Cumulative Array"=w305, "Input Real Time Array"=w306) -> ("Cumulative - Depth vs.Drive Rate"=→"Cumulative - Depth vs. Drive":cluster{dbl[], dbl[]}, "Cumulative - Depth vs. Ik"=→"Cumulative - Depth vs. Ik":cluster{dbl[], dbl[]}, "Real Time - Depth vs. Drive Rate"=→"Real Time - Depth vs. Drive" →"Real Time - Depth vs. Drive":cluster{dbl[], dbl[]}, "Real Time - Depth vs. Ik"=→"Real Time - Depth vs. lk" →"Real Time - Depth vs. lk":cluster{dbl[], dbl[]}, "Current Ik"=w296:dbl, "Depth Rate"=w295:dbl)  [unwired: 2 in]
                n210 = flat-sequence {
                  tunnel: w295 -> [w323]
                  frame #0 {
                    n211 = Multiply(x=w323, y=100) -> (x*y=→"Drive Rate":dbl)
                  }
                }
                n212 = flat-sequence {
                  tunnel: w296 -> [w316]
                  frame #0 {
                    "Ik" <- w316
                    "Ik" <- w316
                  }
                }
              }
              frame 2 {
                n213 = flat-sequence {
                  tunnel: w335 -> [w339]
                  frame #0 {
                    n214 = local read "Output File Slug Test"() -> (w338:path)
                    n215 = call "Slug Test.vi"("# SS"=w339, "Output File"=w338) -> ()  [unwired: 10 in]
                  }
                }
              }
              frame 3 {
                n216 = flat-sequence {
                  tunnel: w343 -> [w353]
                  tunnel: w342 -> [w352]
                  tunnel: w341 -> [w351]
                  tunnel: [w350] -> w340
                  frame #0 {
                    n217 = call "Capture YSI.vi"("Initialize"=w352, "Finished In"=w351, "DEPTH"=w353, "YSI Com Port"="YSI Com Port", "Time Out (secs)"="YSI Time Out (secs)", "Collect Ion Data"="ISE") -> ("Finished Out"=w350:bool)  [unwired: 9 in]
                  }
                }
              }
              frame 4 {
              }
              frame 5 {
                n218 = global read "Global_SIM_switch.vi" "enable_YSI_file"() -> (w359:bool)
                n219 = case shown="True" w359 {
                  tunnel: w361 -> [_ w368]
                  tunnel: w360 -> [_ w367]
                  frame False {
                  }
                  frame True {
                    # "Capture Head Pressure"
                    n220 = local read "Output File YSI Test"() -> (w366:path)
                    n221 = call "Write YSI Data X.vi"("Output File"=w366, "Absolute Depth In"=w367, "Zeroed Pressure"=w368, "Update Pressure = False\nUpdate YSI = True"=FALSE) -> ()  [unwired: 12 in]
                  }
                }
              }
            }
          }
        }
      }
    }
  }
